vi "debug info txt.vi"(2 "data":variant) -> ()   [LabVIEW 2013]
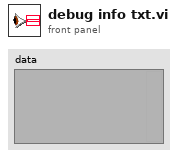
[diagram p1: front panel]
types:
  T1 = enum16{"open", "replace", "create", "open or create", "replace or create", "replace or create with confirmation"}
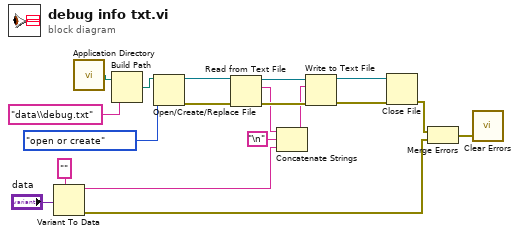
[diagram p0: block diagram]
diagram:
  n1 = Variant To Data(type="" ("字符串"), Variant="data") -> (data=w7:string, error out=w5:errorcluster)  [unwired: 1 in]
  n2 = call <vilib>:"Application Directory.vi"() -> ("Application Directory"=w2:path)
  n3 = Build Path(base path=w2, name or relative path="data\\debug.txt" ("名称或相对路径")) -> (appended path=w3:path)
  n4 = Open/Create/Replace File(file path (use dialog)=w3, operation (0:open)=T1."open or create" ("操作(0:open)")) -> (refnum out=w18:refnum<file>, error out=w17:errorcluster)  [unwired: 4 in, 1 out]
  n5 = Read from Text File(file (use dialog)=w18, error in=w17) -> (refnum out=w16:refnum<file>, text=w14:string, error out=w15:errorcluster)  [unwired: 2 in, 1 out]
  n6 = Concatenate Strings(w14, "\n", w7) -> (w12:string)
  n7 = Write to Text File(file (use dialog)=w16, text=w12, error in=w15) -> (refnum out=w11:refnum<file>, error out=w10:errorcluster)  [unwired: 1 in, 1 out]
  n8 = Close File(refnum=w11, error in=w10) -> (error out=w6:errorcluster)  [unwired: 1 out]
  n9 = Merge Errors(w6, w5) -> (w4:errorcluster)
  n10 = call <vilib>:"Clear Errors.vi"("error in (no error)"=w4) -> ()  [unwired: 6 in, 1 out]
